vi "Attenuator VNA Cannot Support Measurement Warning.vi"(5 "Current Stimulus":T1={"ATT Stimulus"={"Normalize"=TRUE, "Value (dB)"=0.0}, "VNA Stimulus"={"Use Instrument Settings"=FALSE, "Blank Frequencies"=FALSE, "Sweep Type"=enum."Linear", "Sweep"={"Fstart"=500.0, "Fstop"=1500.0, "Units"=enum."MHz", "Points"=201}, "Power (dBm)"=999.0, "IFBW (Hz)"=-1.0, "Sweep Time (s)"=-1.0, "Calibration"={"State"=FALSE, "String"=""}}} {"VNA Stimulus"."Sweep Time (s)" format="%.3g"}, 7 "Requested Stimulus":T1={"ATT Stimulus"={"Normalize"=TRUE, "Value (dB)"=0.0}, "VNA Stimulus"={"Use Instrument Settings"=FALSE, "Blank Frequencies"=FALSE, "Sweep Type"=enum."Linear", "Sweep"={"Fstart"=500.0, "Fstop"=1500.0, "Units"=enum."MHz", "Points"=201}, "Power (dBm)"=999.0, "IFBW (Hz)"=-1.0, "Sweep Time (s)"=-1.0, "Calibration"={"State"=FALSE, "String"=""}}} {"VNA Stimulus"."Sweep Time (s)" format="%.3g"}, 8 "error in (no error)":errorcluster, 11 "Instrument IDN String (\"\")":string) -> (0 "error out":errorcluster, 3 "Choice":T6=enum."Restore")   [LabVIEW 2011]
uses:
  TypeDefs/Attenuator Dialog Response.ctl
  TypeDefs/Attenuator Stimulus Parameters.ctl
  TypeDefs/Attenuator ATT Stimulus.ctl
  TypeDefs/Attenuator VNA Stimulus.ctl
  S Parameter/TypeDefs/SP Frequency Units.ctl
  TypeDefs/Attenuator VNA Calibration State.ctl
  S Parameter/TypeDefs/SP Dialog Response.ctl
panel:
  in  "Abort All":bool
  in  "Abort":bool
  in  "Ignore":bool
  out "Message (\"\")":string="The instrument, %s,  does not support the requested stimulus parameters.  Spartan has set the instrument stimulus parameters as close to the requested values as possible.\n\nPlease select one of the following options:\n\n    Ignore  -  continue with the current stimulus parameters\n    Abort  -  abort this test step\n    Abort All  -  abort the entire sequence"
  out "Cur. Sweep Time":string="0.000"
  out "Req. Sweep Time":string="0.000" caption="Sweep Time"
  out "Sweep Time":cluster{"Pass":bool, "Fail":bool}={"Pass"=TRUE, "Fail"=FALSE}
  out "Cur. IFBW":string="0"
  out "Req. IFBW":string="0" caption="IFBW"
  out "IFBW":cluster{"Pass":bool, "Fail":bool}={"Pass"=TRUE, "Fail"=FALSE}
  out "Cur. Power":string="0"
  out "Req. Power":string="0" caption="Power"
  out "Power":cluster{"Pass":bool, "Fail":bool}={"Pass"=TRUE, "Fail"=FALSE}
  out "Cur. Points":string="0"
  out "Req. Points":string="0" caption="Number of Points"
  out "Points":cluster{"Pass":bool, "Fail":bool}={"Pass"=TRUE, "Fail"=FALSE}
  out "Cur. Stop Freq.":string="0.000"
  out "Req. Stop Freq.":string="0.000" caption="Stop Frequency"
  out "Stop Freq":cluster{"Pass":bool, "Fail":bool}={"Pass"=TRUE, "Fail"=FALSE}
  out "Cur. Start Freq.":string="0.000"
  out "Req. Start Freq.":string="0.000" caption="Start Fequency"
  out "Start Freq":cluster{"Pass":bool, "Fail":bool}={"Pass"=TRUE, "Fail"=FALSE}
  out "Cur. Sweep Type":string="Linear"
  out "Req. Sweep Type":string="Linear" caption="Sweep Type"
  out "Sweep Type":cluster{"Pass":bool, "Fail":bool}={"Pass"=TRUE, "Fail"=FALSE}
  # "Requested"
  # "Current"
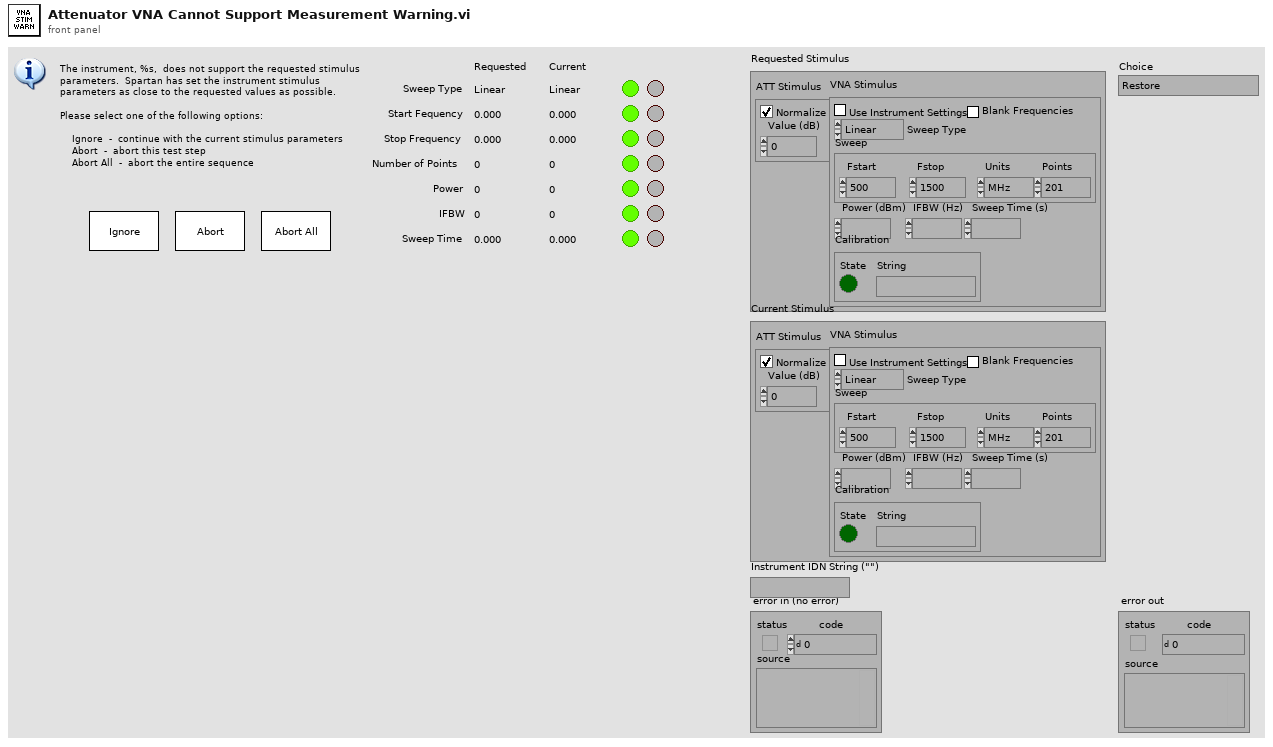
[diagram p1: front panel]
types:
  T1 = typedef "Attenuator Stimulus Parameters.ctl" = cluster{"ATT Stimulus":T2, "VNA Stimulus":T3}
  T2 = typedef "Attenuator ATT Stimulus.ctl" = cluster{"Normalize":bool, "Value (dB)":dbl}
  T3 = typedef "Attenuator VNA Stimulus.ctl" = cluster{"Use Instrument Settings":bool, "Blank Frequencies":bool, "Sweep Type":enum32{"Linear", "Logarithmic", "List", "Power", "CW"}, "Sweep":cluster{"Fstart":dbl, "Fstop":dbl, "Units":T4, "Points":i32}, "Power (dBm)":dbl, "IFBW (Hz)":dbl, "Sweep Time (s)":dbl, "Calibration":T5}
  T4 = typedef "SP Frequency Units.ctl" = enum16{"Hz", "kHz", "MHz", "GHz", "Points"}
  T5 = typedef "Attenuator VNA Calibration State.ctl" = cluster{"State":bool, "String":string}
  T6 = typedef "Attenuator Dialog Response.ctl" = enum16{"None", "Calibrate", "Restore", "Ignore", "Abort", "Abort All"}
  T7 = enum32{"Linear", "Logarithmic", "List", "Power", "CW"}
  T8 = typedef "SP Dialog Response.ctl" = enum16{"None", "Calibrate", "Restore", "Ignore", "Abort", "Abort All"}
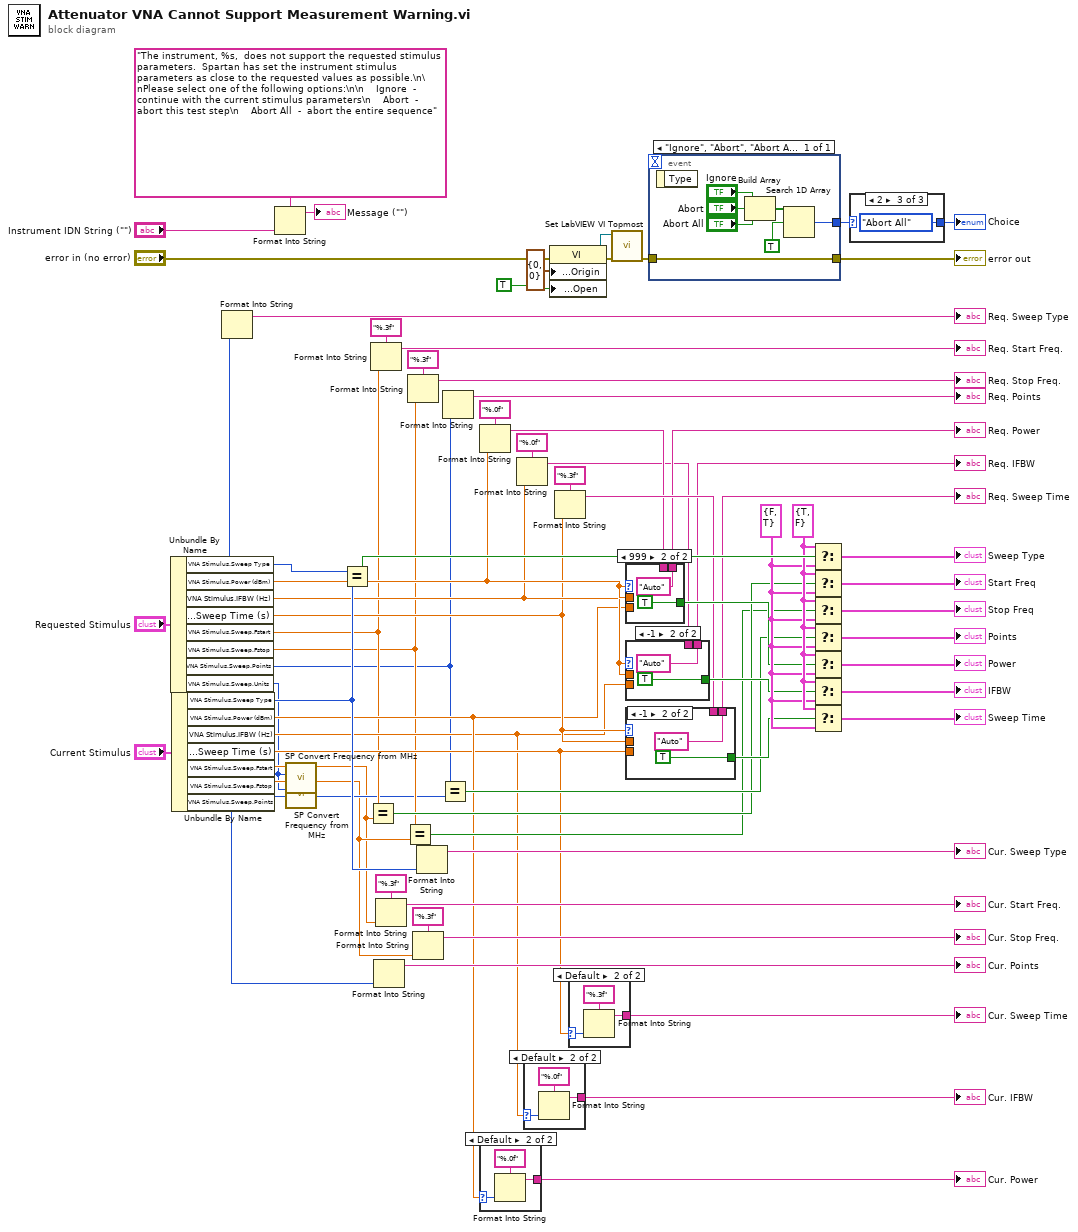
[diagram p0: block diagram]
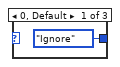
[diagram p2: hidden frame]
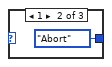
[diagram p3: hidden frame]
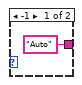
[diagram p4: hidden frame]
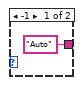
[diagram p5: hidden frame]
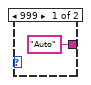
[diagram p6: hidden frame]
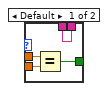
[diagram p7: hidden frame]
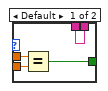
[diagram p8: hidden frame]
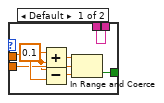
[diagram p9: hidden frame]
diagram:
  w53 = cluster{"Pass":bool, "Fail":bool} {"Pass"=FALSE, "Fail"=TRUE} ("Sweep Type")
  w54 = cluster{"Pass":bool, "Fail":bool} {"Pass"=TRUE, "Fail"=FALSE} ("Sweep Type")
  n1 = Unbundle By Name("Requested Stimulus") -> ("VNA Stimulus.Sweep Type"=w65:T7, "VNA Stimulus.Power (dBm)"=w40:dbl, "VNA Stimulus.IFBW (Hz)"=w38:dbl, "VNA Stimulus.Sweep Time (s)"=w36:dbl, "VNA Stimulus.Sweep.Fstart"=w11:dbl, "VNA Stimulus.Sweep.Fstop"=w10:dbl, "VNA Stimulus.Sweep.Points"=w9:i32, "VNA Stimulus.Sweep.Units"=w3:T4)
  n2 = Unbundle By Name("Current Stimulus") -> ("VNA Stimulus.Sweep Type"=w62:T7, "VNA Stimulus.Power (dBm)"=w23:dbl, "VNA Stimulus.IFBW (Hz)"=w19:dbl, "VNA Stimulus.Sweep Time (s)"=w22:dbl, "VNA Stimulus.Sweep.Fstart"=w7:dbl, "VNA Stimulus.Sweep.Fstop"=w6:dbl, "VNA Stimulus.Sweep.Points"=w8:i32)
  n3 = Format Into String(w65) -> (resulting string=→"Req. Sweep Type":string)  [unwired: 3 in, 1 out]
  n4 = Format Into String(format string="The instrument, %s,  does not support the requested stimulus parameters.  Spartan has set the instrument stimulus parameters as close to the requested values as possible.\n\nPlease select one of the following options:\n\n    Ignore  -  continue with the current stimulus parameters\n    Abort  -  abort this test step\n    Abort All  -  abort the entire sequence", "Instrument IDN String (\"\")") -> (resulting string=→"Message (\"\")":string)  [unwired: 2 in, 1 out]
  n5 = call "SP Convert Frequency from MHz.vi"("Units"=w3, "Frequency (MHz)"=w7) -> ("Converted Frequency"=w4:dbl)  [unwired: 1 in, 8 out]
  n6 = call "SP Convert Frequency from MHz.vi"("Units"=w3, "Frequency (MHz)"=w6) -> ("Converted Frequency"=w5:dbl)  [unwired: 1 in, 8 out]
  n7 = Equal?(x=w65, y=w62) -> (x = y?=w64:bool)
  n8 = Equal?(x=w11, y=w4) -> (x = y?=w48:bool)
  n9 = Format Into String(format string="%.3f", w11) -> (resulting string=→"Req. Start Freq.":string)  [unwired: 2 in, 1 out]
  n10 = Format Into String(w8) -> (resulting string=→"Cur. Points":string)  [unwired: 3 in, 1 out]
  n11 = Format Into String(format string="%.3f", w4) -> (resulting string=→"Cur. Start Freq.":string)  [unwired: 2 in, 1 out]
  n12 = Equal?(x=w10, y=w5) -> (x = y?=w47:bool)
  n13 = Format Into String(format string="%.3f", w10) -> (resulting string=→"Req. Stop Freq.":string)  [unwired: 2 in, 1 out]
  n14 = Format Into String(format string="%.3f", w5) -> (resulting string=→"Cur. Stop Freq.":string)  [unwired: 2 in, 1 out]
  n15 = Format Into String(w62) -> (resulting string=→"Cur. Sweep Type":string)  [unwired: 3 in, 1 out]
  n16 = Equal?(x=w9, y=w8) -> (x = y?=w49:bool)
  n17 = Format Into String(w9) -> (resulting string=→"Req. Points":string)  [unwired: 3 in, 1 out]
  n18 = Format Into String(format string="%.0f", w40) -> (resulting string=w27:string)  [unwired: 2 in, 1 out]
  n19 = case shown="Default" w23 {
    selector: w23 -> [_ w73]
    tunnel: ["Auto" w74] -> w30
    frame 999 {
    }
    frame Default {
      n20 = Format Into String(format string="%.0f", w73) -> (resulting string=w74:string)  [unwired: 2 in, 1 out]
    }
  }
  "Cur. Power" <- w30
  n21 = Format Into String(format string="%.0f", w38) -> (resulting string=w25:string)  [unwired: 2 in, 1 out]
  n22 = case shown="Default" w19 {
    selector: w19 -> [_ w77]
    tunnel: ["Auto" w78] -> w20
    frame -1 {
    }
    frame Default {
      n23 = Format Into String(format string="%.0f", w77) -> (resulting string=w78:string)  [unwired: 2 in, 1 out]
    }
  }
  "Cur. IFBW" <- w20
  n24 = property on="Property Node" class="VI"(error in="error in (no error)", "Front Panel Window:Origin"=cluster{"Horizontal":i16, "Vertical":i16} {"Horizontal"=0, "Vertical"=0}, "Front Panel Window:Open"=TRUE) -> (reference out=w16:refnum<vi>, error out=w17:errorcluster)  [unwired: 1 in]
  n25 = Format Into String(format string="%.3f", w36) -> (resulting string=w29:string)  [unwired: 2 in, 1 out]
  n26 = case shown="Default" w22 {
    selector: w22 -> [_ w81]
    tunnel: ["Auto" w82] -> w21
    frame -1 {
    }
    frame Default {
      n27 = Format Into String(format string="%.3f", w81) -> (resulting string=w82:string)  [unwired: 2 in, 1 out]
    }
  }
  "Cur. Sweep Time" <- w21
  n28 = call "Set LabVIEW VI Topmost.vi"("error in (no error)"=w17, "VI Refnum (null)"=w16) -> ("error out"=w69:errorcluster)  [unwired: 7 in, 2 out]
  n29 = case shown="999" w40 {
    tunnel: w40 -> [w87 _]
    tunnel: w23 -> [w86 _]
    tunnel: [w85 TRUE] -> w52
    tunnel: w27 -> [w84 _]
    tunnel: [w84 "Auto" ("format string")] -> w26
    frame Default {
      n30 = Equal?(x=w87, y=w86) -> (x = y?=w85:bool)
    }
    frame 999 {
    }
  }
  "Req. Power" <- w26
  n31 = case shown="-1" w38 {
    tunnel: w38 -> [w93 _]
    tunnel: w19 -> [w92 _]
    tunnel: [w91 TRUE] -> w51
    tunnel: w25 -> [w90 _]
    tunnel: [w90 "Auto" ("format string")] -> w24
    frame Default {
      n32 = Equal?(x=w93, y=w92) -> (x = y?=w91:bool)
    }
    frame -1 {
    }
  }
  "Req. IFBW" <- w24
  n33 = case shown="-1" w36 {
    tunnel: w36 -> [w96 _]
    tunnel: w22 -> [w97 _]
    tunnel: [w99 TRUE] -> w50
    tunnel: w29 -> [w98 _]
    tunnel: [w98 "Auto" ("format string")] -> w28
    frame Default {
      w100 = 0.1
      n34 = Add(x=w100, y=w96) -> (x+y=w102:dbl)
      n35 = Subtract(x=w96, y=w100) -> (x-y=w101:dbl)
      n36 = In Range and Coerce(upper limit=w102, x=w97, lower limit=w101) -> (In Range?=w99:bool)  [unwired: 1 out]
    }
    frame -1 {
    }
  }
  "Req. Sweep Time" <- w28
  n37 = event shown="[0] \"Ignore\", \"Abort\", \"Abort All\": Value Change" {
    selector: _ -> [_]
    dyn-events: _ -> [_]
    timeout: _ -> [_]
    tunnel: w69 -> [w111]
    tunnel: [w111] -> w71
    tunnel: [w106] -> w2
    event "Ignore", "Abort", "Abort All": Value Change {
      n38 = event-data() -> ()  [unwired: 2 out]
      n39 = Build Array("Ignore", "Abort", "Abort All") -> (w108:bool[])
      n40 = Search 1D Array(1D array=w108, element=TRUE) -> (index of element=w106:i32)  [unwired: 1 out]
    }
  }
  "error out" <- w71
  n41 = Select(t=w54, s=w64, f=w53) -> (s? t:f=→"Sweep Type":cluster{"Pass":bool, "Fail":bool})
  n42 = Select(t=w54, s=w48, f=w53) -> (s? t:f=→"Start Freq":cluster{"Pass":bool, "Fail":bool})
  n43 = Select(t=w54, s=w47, f=w53) -> (s? t:f=→"Stop Freq":cluster{"Pass":bool, "Fail":bool})
  n44 = Select(t=w54, s=w49, f=w53) -> (s? t:f=→"Points":cluster{"Pass":bool, "Fail":bool})
  n45 = Select(t=w54, s=w52, f=w53) -> (s? t:f=→"Power":cluster{"Pass":bool, "Fail":bool})
  n46 = Select(t=w54, s=w51, f=w53) -> (s? t:f=→"IFBW":cluster{"Pass":bool, "Fail":bool})
  n47 = Select(t=w54, s=w50, f=w53) -> (s? t:f=→"Sweep Time":cluster{"Pass":bool, "Fail":bool})
  n48 = case shown="2" w2 {
    tunnel: [SP_Dialog_Response."Ignore" ("Action") SP_Dialog_Response."Abort" ("Action") SP_Dialog_Response."Abort All" ("Action")] -> w1
    frame 0, Default {
    }
    frame 1 {
    }
    frame 2 {
    }
  }
  "Choice" <- w1
